vi "ASCII Stream.vi"() -> ()   [LabVIEW 2019]
uses:
  <vilib>/Instr/_visa.llb/VISA Configure Serial Port (Instr).vi
panel:
  in  "Send":bool
  in  "CMD":string
  out "Chart":dbl(graph)
  out "error out":errorcluster
  in  "stop":bool
  in  "VISA resource name":refnum<visa-resource-name>
  # "Test this VI by first running ASCII Streaming Instrument.vi.  You will need 2 serial ports that are connected via a NULL Modem cable."
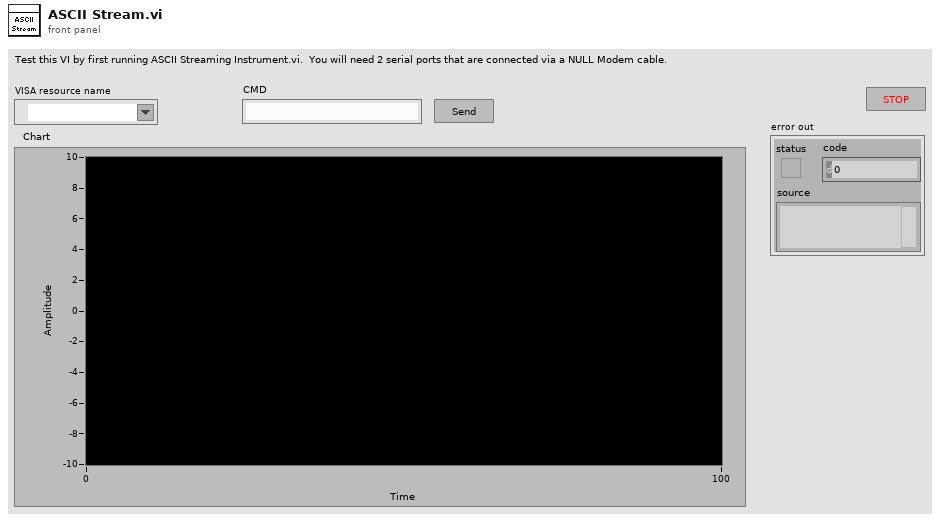
[diagram p1: front panel]
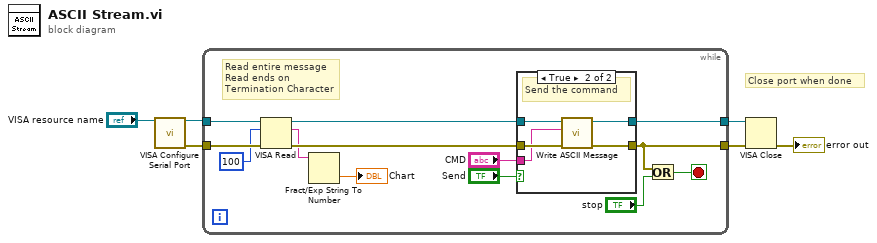
[diagram p0: block diagram]
diagram:
  # "Close port when done"
  n1 = call-poly "VISA Configure Serial Port"("VISA resource name"="VISA resource name") -> ("VISA resource name out"=w1:refnum<visa-resource-name>, "error out"=w4:errorcluster)  [unwired: 13 in]
  n2 = while {
    tunnel: w4 -> [w19]
    tunnel: w1 -> [w16]
    tunnel: [w15] -> w2
    tunnel: [w18] -> w6
    stop <- w14 stop-if-true
    # "Read entire message\nRead ends on\nTermination Character"
    n3 = VISA Read(VISA resource name=w16, byte count=u32 100, error in (no error)=w19) -> (VISA resource name out=w11:refnum<visa-resource-name>, read buffer=w10:string, error out=w17:errorcluster)  [unwired: 1 out]
    n4 = Fract/Exp String To Number(string=w10) -> (number=→"Chart":dbl)  [unwired: 3 in, 1 out]
    n5 = case shown="True" "Send" {
      tunnel: [w21 w26] -> w18
      tunnel: [w20 w24] -> w15
      tunnel: w17 -> [w21 w25]
      tunnel: w11 -> [w20 w23]
      tunnel: "CMD" -> [_ w22]
      frame False {
        # "Do nothing"
      }
      frame True {
        # "Send the command"
        n6 = call "Write ASCII Message.vi"("error in"=w25, "Message"=w22, "VISA resource in"=w23) -> ("error out"=w26:errorcluster, "VISA resource out"=w24:refnum<visa-resource-name>)  [unwired: 7 in]
      }
    }
    n7 = Or(x=w18, y="stop") -> (x .or. y?=w14:bool)
  }
  n8 = VISA Close(VISA resource name=w2, error in (no error)=w6) -> (error out=→"error out":errorcluster)
